vi "Five 8-bit Ports Digital Output.vi"(2 "Packet":u64, 4 "Five 8-bit DO Ports":T1={"8-bit DO Port0"="Chassis1/Mod3/DO7:0", "8-bit DO Port1"="Chassis1/Mod3/DO7:0", "8-bit DO Port2"="Chassis1/Mod3/DO7:0", "8-bit DO Port3"="Chassis1/Mod3/DO7:0", "8-bit DO Port4"="Chassis1/Mod3/DO7:0"}) -> ()   [LabVIEW 2009]
uses:
  <vilib>/eio/EIONode/EIONode.xnode
  <vilib>/rvi/eio/nirviEIOImplementation/nirviEIOImplementation.xnode
  <vilib>/rvi/eio/common/nirviEmuTemplateMethod_noerrors.vi
  <vilib>/rvi/eio/common/nirviEmuClasses.ctl
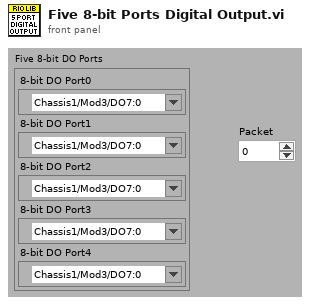
[diagram p1: front panel]
types:
  T1 = cluster{"8-bit DO Port0":refnum<k21>, "8-bit DO Port1":refnum<k21>, "8-bit DO Port2":refnum<k21>, "8-bit DO Port3":refnum<k21>, "8-bit DO Port4":refnum<k21>}
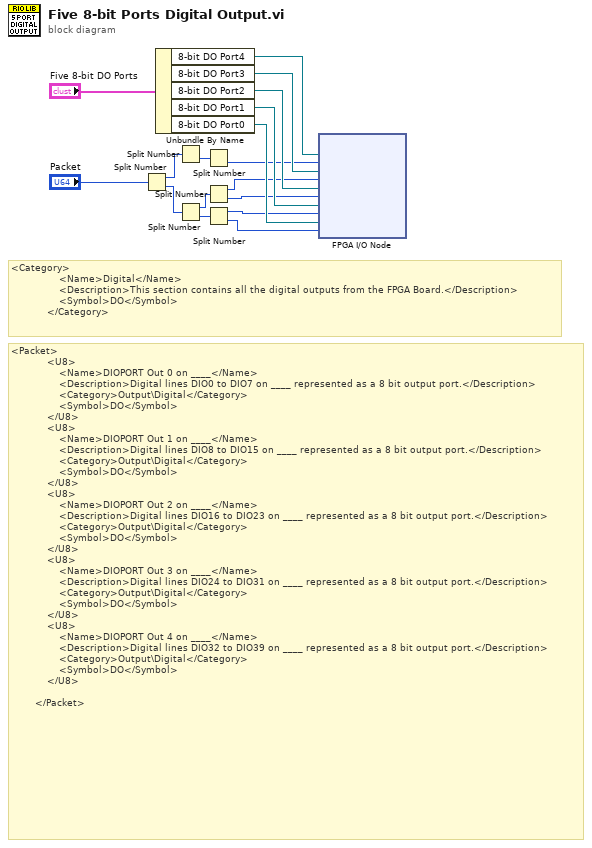
[diagram p0: block diagram]
diagram:
  # "<Packet>\n            <U8>\n                <Name>DIOPORT Out 0 on ____</Name>\n                <Description>Digital lines DIO0 to DIO7 on ____ represented as a 8 bit output port.</Description>\n                <Category>Output\\Digital</Category>\n                <Symbol>DO</Symbol>\n            </U8>\n            <U8>\n                <Name>DIOPORT Out 1 on ____</Name>\n                <Description>Digital lines DIO8 to DIO15 on ____ represented as a 8 bit output port.</Description>\n                <Category>Output\\Digital</Category>\n                <Symbol>DO</Symbol>\n            </U8>\n            <U8>\n                <Name>DIOPORT Out 2 on ____</Name>\n                <Description>Digital lines DIO16 to DIO23 on ____ represented as a 8 bit output port.</Description>\n                <Category>Output\\Digital</Category>\n                <Symbol>DO</Symbol>\n            </U8>\n            <U8>\n                <Name>DIOPORT Out 3 on ____</Name>\n                <Description>Digital lines DIO24 to DIO31 on ____ represented as a 8 bit output port.</Description>\n                <Category>Output\\Digital</Category>\n                <Symbol>DO</Symbol>\n            </U8>\n            <U8>\n                <Name>DIOPORT Out 4 on ____</Name>\n                <Description>Digital lines DIO32 to DIO39 on ____ represented as a 8 bit output port.</Description>\n                <Category>Output\\Digital</Category>\n                <Symbol>DO</Symbol>\n            </U8>\n\n        </Packet>"
  # "<Category>\n                <Name>Digital</Name>\n                <Description>This section contains all the digital outputs from the FPGA Board.</Description>\n                <Symbol>DO</Symbol>\n            </Category>"
  n1 = Split Number(x="Packet") -> (hi(x)=w3:u32, lo(x)=w16:u32)
  n2 = Unbundle By Name("Five 8-bit DO Ports") -> ("8-bit DO Port4"=w4:refnum<k21>, "8-bit DO Port3"=w6:refnum<k21>, "8-bit DO Port2"=w9:refnum<k21>, "8-bit DO Port1"=w12:refnum<k21>, "8-bit DO Port0"=w11:refnum<k21>)
  n3 = Split Number(x=w3) -> (lo(x)=w2:u16)  [unwired: 1 out]
  n4 = Split Number(x=w16) -> (hi(x)=w8:u16, lo(x)=w17:u16)
  n5 = Split Number(x=w2) -> (lo(x)=w1:u8)  [unwired: 1 out]
  n6 = Split Number(x=w8) -> (hi(x)=w5:u8, lo(x)=w7:u8)
  n7 = Split Number(x=w17) -> (hi(x)=w10:u8, lo(x)=w15:u8)
  n8 = xnode "FPGA I/O Node"("I/O Item"=w1, "I/O Item"=w5, "I/O Item"=w7, "I/O Item"=w10, "I/O Item"=w15, "FPGA I/O In"=w4, "FPGA I/O In"=w6, "FPGA I/O In"=w9, "FPGA I/O In"=w12, "FPGA I/O In"=w11) -> ()  [unwired: 5 out]
